vi "from string.vi"(8 "error in":errorcluster, 9 "data":string, 10 "version":string, 11 "Scan Engine configuration in":refnum<class "Scan Engine configuration.lvclass">) -> (0 "error out":errorcluster, 3 "Scan Engine configuration out":refnum<class "Scan Engine configuration.lvclass">)   [LabVIEW 2015, in "Scan Engine configuration.lvclass"]
doc: "Provides an interface for loading a module configuration from a file or other serialized data source. It is recommended that all children of this class store data in two sets--data required for its own initialization, and any data required for parent initialization--and that each implementation uses the <b>Call Parent Method</b> primitive to de-serialize parent information. As a result, it is expected that every module configuration class calls <b>component configuration.lvclass:From String.vi</b>."
uses:
  Scan Engine configuration.lvclass
  <vilib>/NI/Tag Bus Module Framework/channel/TBM channel.lvclass
  Line.ctl
  Scan Engine configuration.lvclass/Scan Engine configuration.ctl
  <vilib>/NI/Tag Bus Module Framework/module configuration/TBM module configuration.lvclass
  <vilib>/NI/Configuration Framework/serializable configuration/NISE_CEF_serializable configuration.lvclass
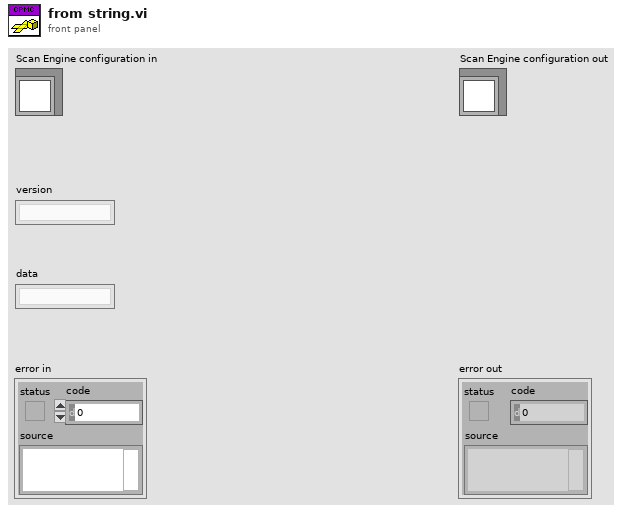
[diagram p1: front panel]
types:
  T1 = typedef "Scan Engine configuration.lvclass/Line.ctl" = cluster{"channel":refnum<class "TBM channel.lvclass">, "Tag":string}
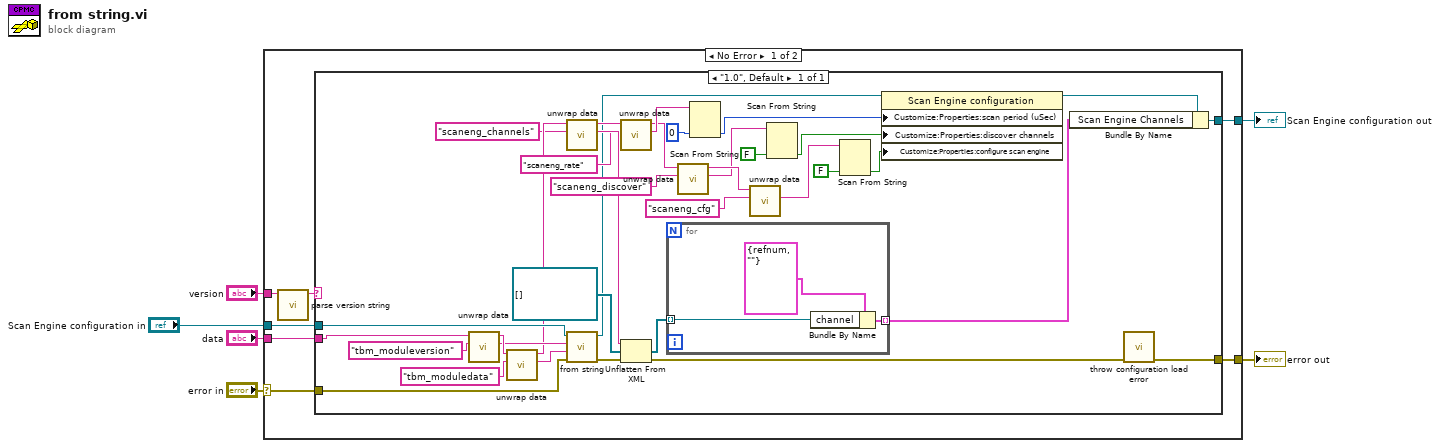
[diagram p0: block diagram]
diagram:
  n1 = case shown="No Error" "error in" {
    selector: "error in" -> [w7 w53]
    tunnel: "data" -> [w13 _]
    tunnel: "Scan Engine configuration in" -> [w12 w52]
    tunnel: [w11 w52] -> w5
    tunnel: [w10 w53] -> w4
    tunnel: "version" -> [w9 _]
    frame No Error {
      n2 = call <vilib>:"parse version string.vi"("full version"=w9) -> ("major.minor version"=w8:string)  [unwired: 7 in, 3 out]
      n3 = case shown="\"1.0\", Default" w8 {
        tunnel: w13 -> [w45]
        tunnel: w7 -> [w44]
        tunnel: w12 -> [w48]
        tunnel: [w37] -> w11
        tunnel: [w47] -> w10
        frame "1.0", Default {
          n4 = call <vilib>:"unwrap data.vi"("identifier"="tbm_moduleversion" ("additional identifier"), "data to unwrap"=w45) -> ("unwrapped data"=w40:string, "remaining string"=w46:string)  [unwired: 8 in]
          n5 = call <vilib>:"unwrap data.vi"("identifier"="tbm_moduledata" ("additional identifier"), "data to unwrap"=w46) -> ("unwrapped data"=w42:string, "remaining string"=w39:string)  [unwired: 8 in]
          n6 = call <vilib>:"unwrap data.vi"("identifier"="scaneng_channels" ("additional identifier"), "data to unwrap"=w39) -> ("unwrapped data"=w36:string, "remaining string"=w32:string)  [unwired: 8 in]
          n7 = call-parent "from string.vi"("error in"=w44, "data"=w42, "version"=w40, "module configuration in"=w48) -> ("error out"=w35:errorcluster, "module configuration out"=w29:refnum<class "Scan Engine configuration.lvclass">)  [unwired: 6 in]
          n8 = call <vilib>:"unwrap data.vi"("identifier"="scaneng_rate" ("additional identifier"), "data to unwrap"=w32) -> ("unwrapped data"=w26:string, "remaining string"=w25:string)  [unwired: 8 in]
          n9 = Unflatten From XML(xml string=w36, type=refnum<class "TBM channel.lvclass">[] [] ("Lines"), error in (no error)=w35) -> (value=w15:refnum<class "TBM channel.lvclass">[], error out=w34:errorcluster)
          n10 = for {
            tunnel: w15 -> [w50] mode=indexing
            tunnel: [w49] -> w14 mode=indexing
            n11 = Bundle By Name(cluster=T1 {"channel"=refnum, "Tag"=""} ("Line"), "channel"=w50) -> (w49:T1)
          }
          n12 = call <vilib>:"unwrap data.vi"("identifier"="scaneng_discover" ("additional identifier"), "data to unwrap"=w25) -> ("unwrapped data"=w22:string, "remaining string"=w23:string)  [unwired: 8 in]
          n13 = Scan From String(input string=w26, default 1=u32 0 ("default value 1")) -> (output 1=w28:u32)  [unwired: 3 in, 3 out]
          n14 = call <vilib>:"unwrap data.vi"("identifier"="scaneng_cfg" ("additional identifier"), "data to unwrap"=w23) -> ("unwrapped data"=w18:string)  [unwired: 8 in, 1 out]
          n15 = Scan From String(input string=w22, default 1=FALSE) -> (output 1=w20:bool)  [unwired: 3 in, 3 out]
          n16 = Scan From String(input string=w18, default 1=FALSE) -> (output 1=w17:bool)  [unwired: 3 in, 3 out]
          n17 = property class="Scan Engine configuration"(reference=w29, "Customize:Properties:scan period (uSec)"=w28, "Customize:Properties:discover channels"=w20, "Customize:Properties:configure scan engine"=w17) -> (reference out=w16:refnum<class "Scan Engine configuration.lvclass">)  [unwired: 1 in, 1 out]
          n18 = Bundle By Name(cluster=w16, "Scan Engine Channels"=w14) -> (w37:refnum<class "Scan Engine configuration.lvclass">)
          n19 = call <vilib>:"throw configuration load error.vi"("error in"=w34) -> ("error out"=w47:errorcluster)  [unwired: 10 in]
        }
      }
    }
    frame Error {
    }
  }
  "error out" <- w4
  "Scan Engine configuration out" <- w5
